vi "AndorShutdown.vi"(5 "ShutDownRef":refnum<vi>, 7 "CurrentTempRef":refnum<vi>, 8 "error in":errorcluster, 10 "CoolerON":bool, 11 "SetTemp":bool) -> (0 "error out":errorcluster, 2 "ShutDown":cluster{"CoolOff":bool, "ShutDown":bool}, 3 "CurrentTemp":i32)   [LabVIEW 2014]
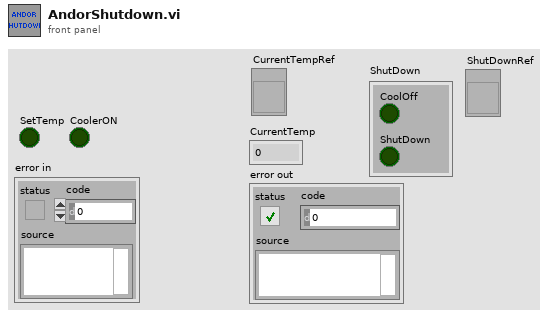
[diagram p1: front panel]
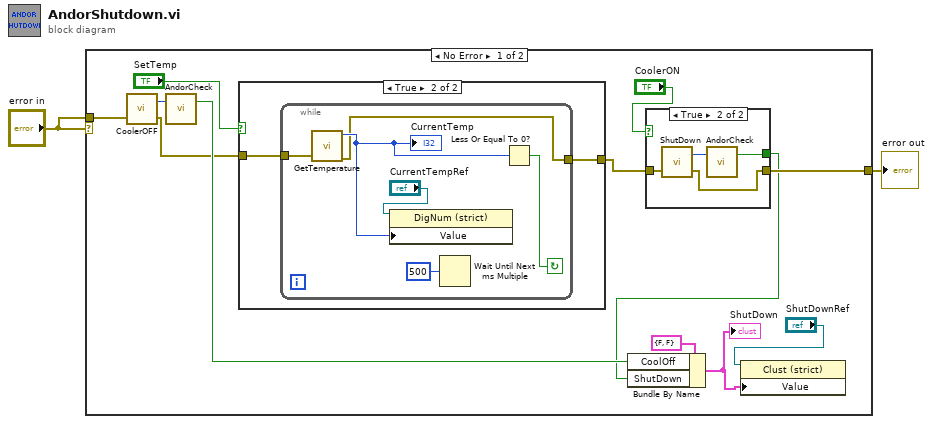
[diagram p0: block diagram]
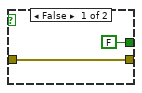
[diagram p2: hidden frame]
diagram:
  n1 = case shown="No Error" "error in" {
    tunnel: "error in" -> [w14 w30]
    tunnel: [w9 w30] -> w1
    frame No Error {
      n2 = call <userlib>:"CoolerOFF.vi"("error in (no error)"=w14) -> ("error out"=w3:errorcluster, "DLL error code"=w13:u32)  [unwired: 1 in]
      n3 = call "AndorCheck.vi"("Input"=w13) -> ("Status"=w5:bool)  [unwired: 1 in, 1 out]
      n4 = case shown="True" "SetTemp" {
        tunnel: w3 -> [w21 w23]
        tunnel: [w21 w22] -> w10
        frame False {
        }
        frame True {
          n5 = while {
            tunnel: w23 -> [w29]
            tunnel: [w24] -> w22
            stop <- w26 continue-if-true
            n6 = call <userlib>:"GetTemperature.vi"("error in (no error)"=w29) -> ("error out"=w24:errorcluster, "temperature"=w27:i32)  [unwired: 3 in, 2 out]
            "CurrentTemp" <- w27
            n7 = property class="DigNum (strict)"(reference="CurrentTempRef", "Value"=w27) -> ()  [unwired: 1 in, 2 out]
            n8 = Wait Until Next ms Multiple(millisecond multiple=u32 500) -> ()  [unwired: 1 out]
            n9 = Less Or Equal To 0?(x=w27) -> (x <= 0?=w26:bool)
          }
        }
      }
      n10 = case shown="True" "CoolerON" {
        tunnel: w10 -> [w16 w20]
        tunnel: [FALSE ("Status") w18] -> w4
        tunnel: [w16 w17] -> w9
        frame False {
        }
        frame True {
          n11 = call <userlib>:"ShutDown.vi"("error in (no error)"=w20) -> ("error out"=w17:errorcluster, "DLL error code"=w19:u32)  [unwired: 1 in]
          n12 = call "AndorCheck.vi"("Input"=w19) -> ("Status"=w18:bool)  [unwired: 1 in, 1 out]
        }
      }
      n13 = Bundle By Name(cluster=cluster{"CoolOff":bool, "ShutDown":bool} {"CoolOff"=FALSE, "ShutDown"=FALSE} ("ShutDown"), "CoolOff"=w5, "ShutDown"=w4) -> (w6:cluster{"CoolOff":bool, "ShutDown":bool})
      "ShutDown" <- w6
      n14 = property class="Clust (strict)"(reference="ShutDownRef", "Value"=w6) -> ()  [unwired: 1 in, 2 out]
    }
    frame Error {
    }
  }
  "error out" <- w1
